vi "Measure Range Select.vi"(8 "error in (no error)":errorcluster, 10 "Range Select":enum16{"200mV", "2V", "20V", "200V", "1000V"}(ring), 11 "VISA resource name":refnum<visa-resource-name>) -> (0 "error out":errorcluster, 2 "Numeric":dbl, 3 "VISA resource out":refnum<visa-resource-name>)   [LabVIEW 2020]
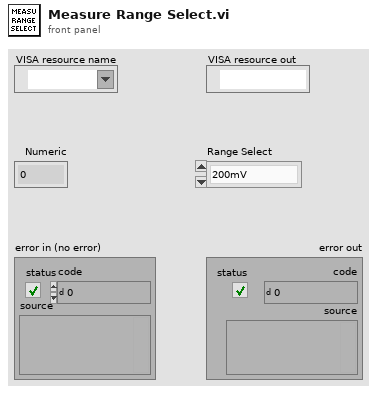
[diagram p1: front panel]
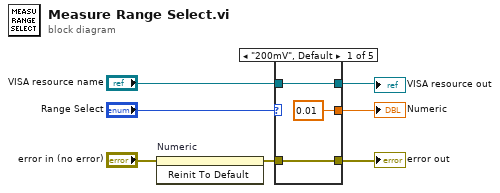
[diagram p0: block diagram]
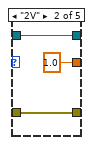
[diagram p2: hidden frame]
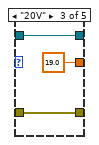
[diagram p3: hidden frame]
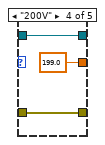
[diagram p4: hidden frame]
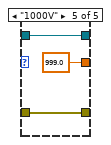
[diagram p5: hidden frame]
diagram:
  n1 = invoke on="Numeric" class="DigNum (strict)" method="Reinit To Default"(error in="error in (no error)") -> (error out=w3:errorcluster)  [unwired: 2 in, 2 out]
  n2 = case shown="\"200mV\", Default" "Range Select" {
    tunnel: [0.01 1.0 19.0 199.0 999.0] -> w6
    tunnel: [w9 w12 w15 w18 w21] -> w4
    tunnel: w3 -> [w9 w12 w15 w18 w21]
    tunnel: "VISA resource name" -> [w8 w11 w14 w17 w20]
    tunnel: [w8 w11 w14 w17 w20] -> w1
    frame "200mV", Default {
    }
    frame "2V" {
    }
    frame "20V" {
    }
    frame "200V" {
    }
    frame "1000V" {
    }
  }
  "Numeric" <- w6
  "error out" <- w4
  "VISA resource out" <- w1
